vi "Create Message Queue.vi"(8 "Error In":errorcluster) -> (0 "Error Out":errorcluster)   [LabVIEW 2023, in "QSM - Main.lvlib"]
doc: "This VI creates the message queue for the Queued State Machine template."
uses:
  QSM - Main.lvlib
  Controls/Message Queue Element.ctl
  Controls/State Machine Message.ctl
  Controls/Message Queue Reference Functional Global Variable Operation.ctl
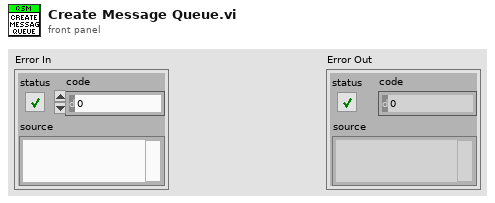
[diagram p1: front panel]
types:
  T1 = typedef "QSM - Main.lvlib/Message Queue Reference Functional Global Variable Operation.ctl" = enum16{"Set", "Get"}
  T2 = typedef "QSM - Main.lvlib/Message Queue Element.ctl" = cluster{"State Machine Message":T3, "Data":variant}
  T3 = typedef "QSM - Main.lvlib/State Machine Message.ctl" = enum16{"Initialize", "Handle Error", "Exit"}
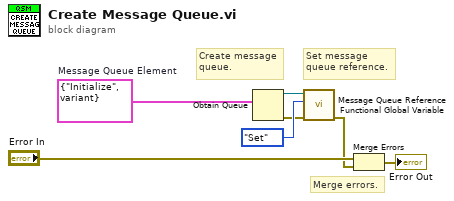
[diagram p0: block diagram]
diagram:
  w7 = T2 {"State Machine Message"=enum."Initialize", "Data"=variant}  # Message Queue Element
  # "Merge errors."
  # "Create message\nqueue."
  # "Set message\nqueue reference."
  n1 = Obtain Queue(element data type=w7) -> (queue out=w5:refnum<queue>, error out=w4:errorcluster)  [unwired: 4 in, 1 out]
  n2 = call "Message Queue Reference Functional Global Variable.vi"("Error In"=w4, "Operation"=Message_Queue_Reference_Functional_Global_Variable_Operation."Set", "Message Queue Reference In"=w5) -> ("Error Out"=w1:errorcluster)  [unwired: 7 in, 1 out]
  n3 = Merge Errors("Error In", w1) -> (→"Error Out":errorcluster)
